vi "Uint32 Destroy.vi"(8 "error in (no error)":errorcluster, 11 "Uint32 DVR in":refnum<data-value>) -> (0 "error out":errorcluster)   [LabVIEW 2012, in "MDSplus.lvlib"]
uses:
  <vilib>/MDSplus/Library/MDSplus.lvlib
  <vilib>/MDSplus/Classes/Data_Class/Scalar_Class/Uint32_Class/Uint32.lvclass
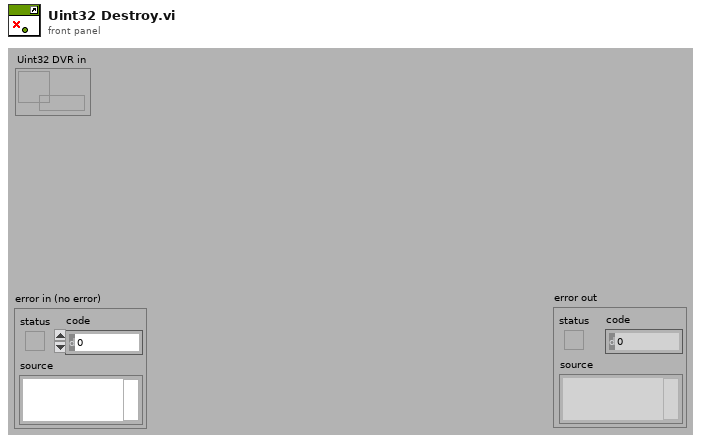
[diagram p1: front panel]
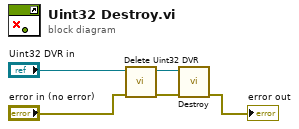
[diagram p0: block diagram]
diagram:
  n1 = call <vilib>:"Delete Uint32 DVR.vi"("error in (no error)"="error in (no error)", "Uint32 DVR in"="Uint32 DVR in") -> ("error out"=w2:errorcluster, "Uint32 out"=w3:refnum<class "Uint32.lvclass">)  [unwired: 8 in]
  n2 = call-dynamic "Destroy.vi"("error in (no error)"=w2, "Uint32 in"=w3) -> ("error out"=→"error out":errorcluster)  [unwired: 9 in]
